vi "Tree_GetTagfromText.vi"(8 "Error In":errorcluster, 10 "Item Text IN":string, 11 "Tree Refnum":refnum<vi>) -> (0 "Error Out":errorcluster, 2 "Item Tag OUT":string, 3 "Tree Refnum 2":refnum<vi>)   [LabVIEW 2012]
doc: "SciScan 1.2 160622"
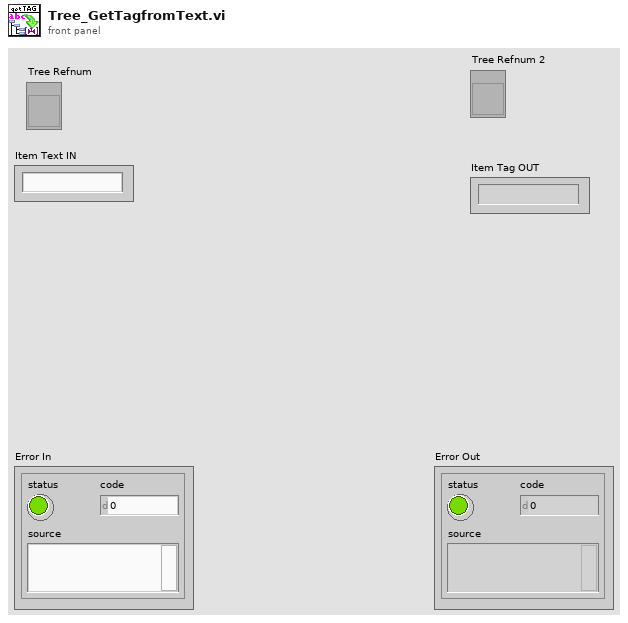
[diagram p1: front panel]
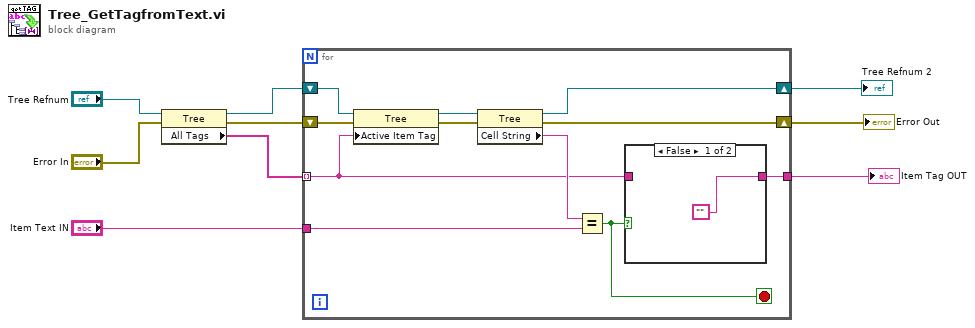
[diagram p0: block diagram]
diagram:
  n1 = property class="Tree"(reference="Tree Refnum", error in="Error In") -> (reference out=w7:refnum<vi>, error out=w6:errorcluster, "All Tags"=w8:string[])
  n2 = for {
    tunnel: w8 -> [w11] mode=indexing
    shift-right: [w16] -> w2
    shift-left: w6 -> [w17]
    shift-right: [w15] -> w1
    shift-left: w7 -> [w20]
    tunnel: "Item Text IN" -> [w14]
    tunnel: [w10] -> w4
    stop <- w12 stop-if-true
    n3 = property class="Tree"(reference=w20, error in=w17, "Active Item Tag"=w11) -> (reference out=w19:refnum<vi>, error out=w18:errorcluster)
    n4 = property class="Tree"(reference=w19, error in=w18) -> (reference out=w15:refnum<vi>, error out=w16:errorcluster, "Cell String"=w13:string)
    n5 = Equal?(x=w13, y=w14) -> (x = y?=w12:bool)
    n6 = case shown="False" w12 {
      tunnel: w11 -> [_ w22]
      tunnel: ["" w22] -> w10
      frame False {
      }
      frame True {
      }
    }
  }
  "Error Out" <- w2
  "Item Tag OUT" <- w4
  "Tree Refnum 2" <- w1
